vi "test - Read CSM Log Filter Config.vi"(8 "error in (no error)":errorcluster, 11 "TestCase in":refnum<class "labview-config-library.lvclass">) -> (0 "error out":errorcluster, 3 "TestCase out":refnum<class "labview-config-library.lvclass">)   [LabVIEW 2017, in "labview-config-library.lvclass"]
uses:
  labview-config-library.lvclass
  <userlib>/_NEVSTOP/Communicable State Machine(CSM)/_Support/Typedef/_CSM_GlobalLog Filter Rules - v1.0.ctl
  <userlib>/_NEVSTOP/Communicable State Machine(CSM)/_Support/Typedef/_CSM_GlobalLog_MSG_TYPE.ctl
  <userlib>/_NEVSTOP/Communicable State Machine(CSM)/_Support/Typedef/_CSM_GlobalLog_STATE_TYPE.ctl
  <vilib>/addons/_JKI Toolkits/VI Tester/TestCase.llb/TestCase.lvclass
  <userlib>/_NEVSTOP/Communicable State Machine(CSM)/Communicable State Machine.lvlib
  C:/Program Files (x86)/National Instruments/LabVIEW 2017/vi.lib/addons/_JKI Toolkits/VI Tester/TestCase.llb/TestCase.lvclass
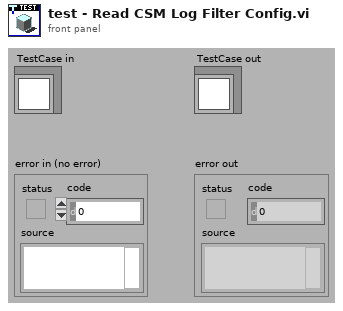
[diagram p1: front panel]
types:
  T1 = typedef "Communicable State Machine.lvlib/_CSM_GlobalLog Filter Rules - v1.0.ctl" = cluster{"Global":cluster{"CSM":string[], "LogType":T2[], "State":string[], "StateType":T3[]}, "CSM":cluster{"LogType":cluster{"CSM":string, "LogType":T2}[], "State":cluster{"CSM":string, "State":string}[], "StateType":cluster{"CSM":string, "LogType":T3}[]}}
  T2 = typedef "Communicable State Machine.lvlib/_CSM_GlobalLog_MSG_TYPE.ctl" = enum16{"User Log", "State Change", "Status", "Interrupt", "Register", "Unregister", "Error Log", "Module Created", "Module Destroyed"}
  T3 = typedef "Communicable State Machine.lvlib/_CSM_GlobalLog_STATE_TYPE.ctl" = enum16{"State - Internal State", "State - External Message", "State - Response", "State - Complete"}
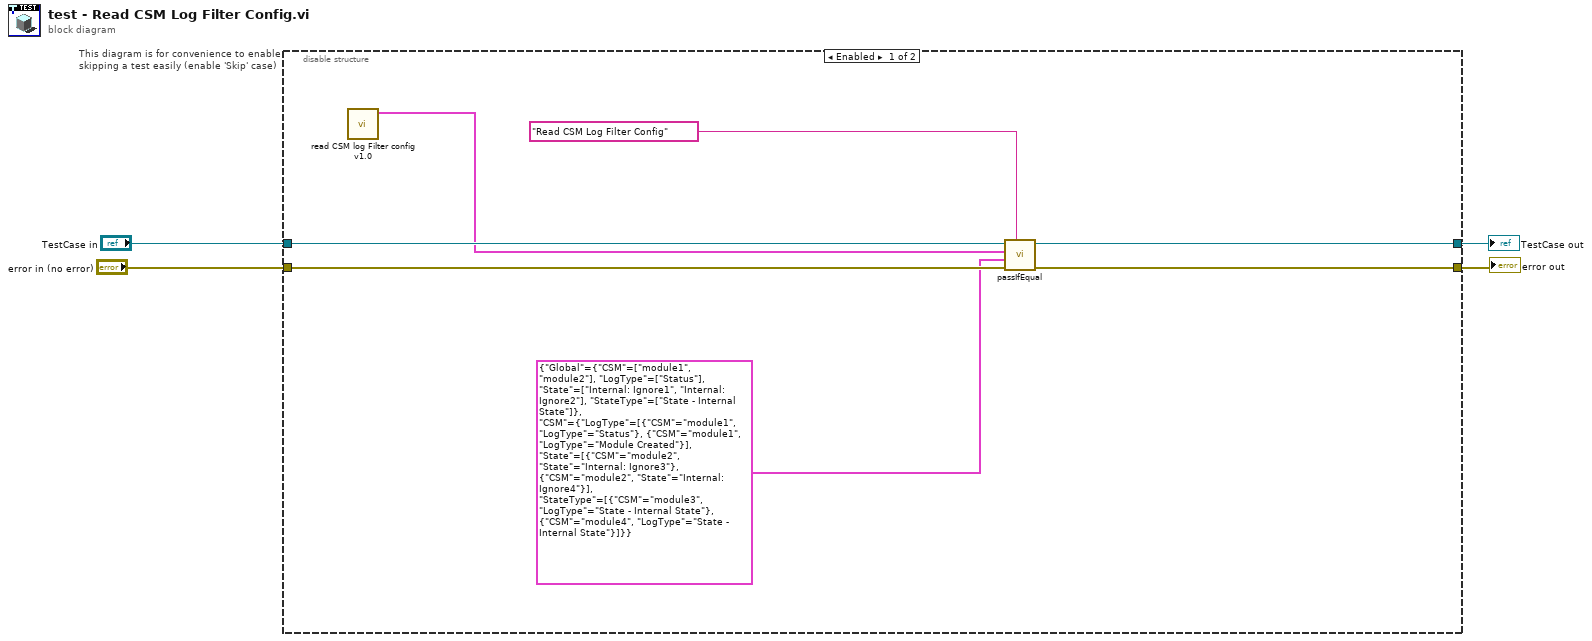
[diagram p0: block diagram]
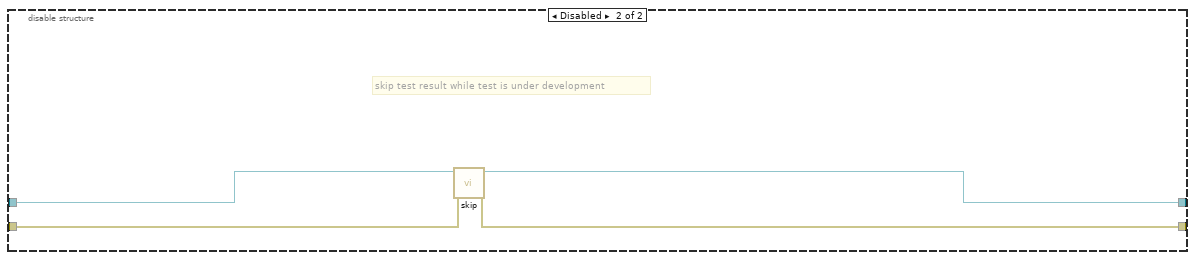
[diagram p2: hidden frame]
diagram:
  n1 = disable-structure "This diagram is for convenience to enable skipping a test easily (enable 'Skip' case)" shown="Enabled" {
    disable-tunnel: "TestCase in" -> [w11 w15]
    disable-tunnel: [w8 w13] -> w1
    disable-tunnel: [w9 w14] -> w3
    disable-tunnel: "error in (no error)" -> [w10 w12]
    frame Enabled {
      n2 = call "read CSM log Filter config v1.0.vi"() -> ("Rules-v1"=w6:T1)  [unwired: 11 in]
      n3 = call-dynamic "passIfEqual.vi"("custom report message (\"\")"="Read CSM Log Filter Config" ("custom report message (\"\")"), "error in (no error)"=w10, "y"=T1 {"Global"={"CSM"=["module1", "module2"], "LogType"=[enum."Status"], "State"=["Internal: Ignore1", "Internal: Ignore2"], "StateType"=[enum."State - Internal State"]}, "CSM"={"LogType"=[{"CSM"="module1", "LogType"=enum."Status"}, {"CSM"="module1", "LogType"=enum."Module Created"}], "State"=[{"CSM"="module2", "State"="Internal: Ignore3"}, {"CSM"="module2", "State"="Internal: Ignore4"}], "StateType"=[{"CSM"="module3", "LogType"=enum."State - Internal State"}, {"CSM"="module4", "LogType"=enum."State - Internal State"}]}} ("Rules-v1"), "x"=w6, "TestCase in"=w11) -> ("error out"=w9:errorcluster, "TestCase out"=w8:refnum<class "labview-config-library.lvclass">)  [unwired: 5 in]
    }
    frame Disabled {
      # "skip test result while test is under development"
      n4 = call <vilib>:"skip.vi"("error in (no error)"=w12, "TestCase in"=w15) -> ("error out"=w14:errorcluster, "TestCase out"=w13:refnum<class "labview-config-library.lvclass">)  [unwired: 8 in]
    }
  }
  "error out" <- w3
  "TestCase out" <- w1
